vi "ID conformity.vi"(10 "项名":string[][](array[string])) -> (2 "ID conformity":string)   [LabVIEW 2020]
panel:
  out "ID":string[](array[string])
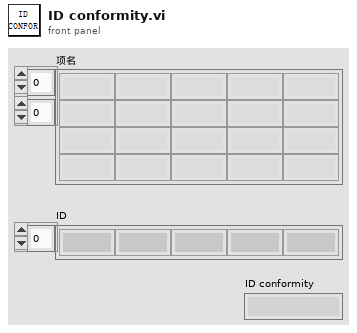
[diagram p1: front panel]
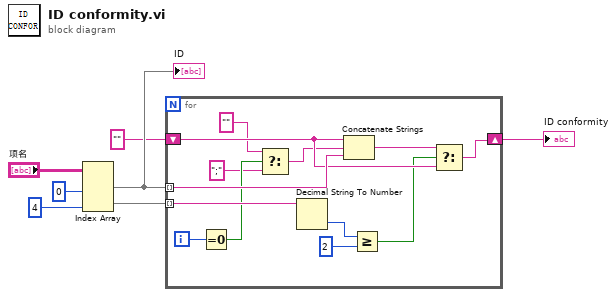
[diagram p0: block diagram]
diagram:
  n1 = Index Array(array="项名", index (col) #1=0 ("禁用的索引 (列)"), index (col) #2=4 ("索引 (列)")) -> (element #1=w4:string[], element #2=w3:string[])  [unwired: 2 in]
  "ID" <- w4
  n2 = for {
    tunnel: w4 -> [w17] mode=indexing
    tunnel: w3 -> [w20] mode=indexing
    shift-right: [w15] -> w2
    shift-left: "" -> [w14]
    i -> [w13]
    n3 = Equal To 0?(x=w13) -> (x = 0?=w12:bool)
    n4 = Select(t="", s=w12, f=";") -> (s? t:f=w9:string)
    n5 = Decimal String To Number(string=w20) -> (number=w19:i32)  [unwired: 2 in, 1 out]
    n6 = Concatenate Strings(w14, w9, w17) -> (w16:string)
    n7 = Greater Or Equal?(x=w19, y=2) -> (x >= y?=w8:bool)
    n8 = Select(t=w16, s=w8, f=w14) -> (s? t:f=w15:string)
  }
  "ID conformity" <- w2
